vi "Read Hardware Interface State.vi"(8 "error in (no error)":errorcluster, 10 "hardware interface index":u16, 11 "PLBB in":refnum<class "PL BlackBox Modbus Client.lvclass">) -> (0 "error out":errorcluster, 2 "hardware interface state":T1, 3 "PLBB out":refnum<class "PL BlackBox Modbus Client.lvclass">)   [LabVIEW 2015, in "PL BlackBox Modbus Client.lvclass"]
doc: "Reads the hardware interface state."
uses:
  PL BlackBox Modbus Client.lvclass
  <vilib>/plasmapper/PL Modbus Client/PL Modbus Client.lvclass
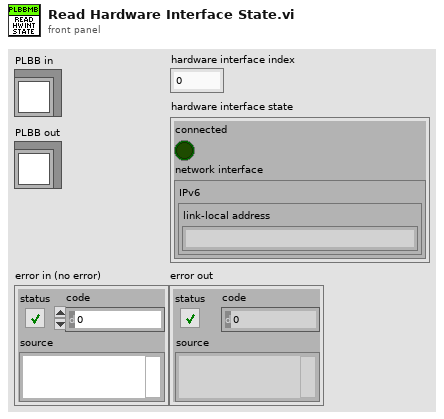
[diagram p1: front panel]
types:
  T1 = cluster{"connected":bool, "network interface":cluster{"IPv6":cluster{"link-local address":string}}}
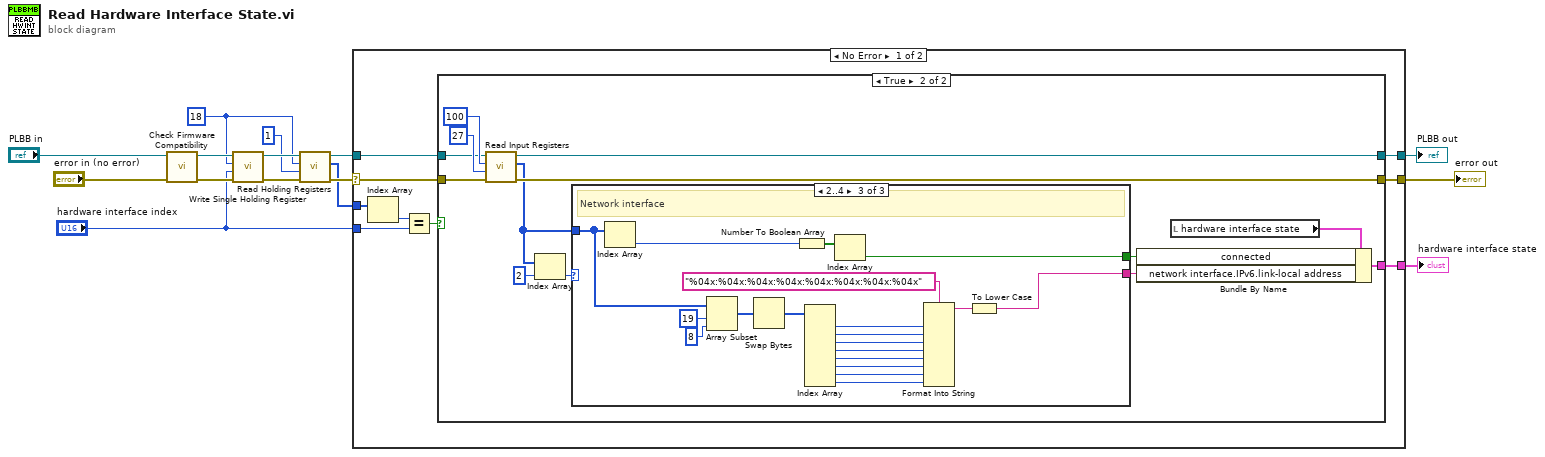
[diagram p0: block diagram]
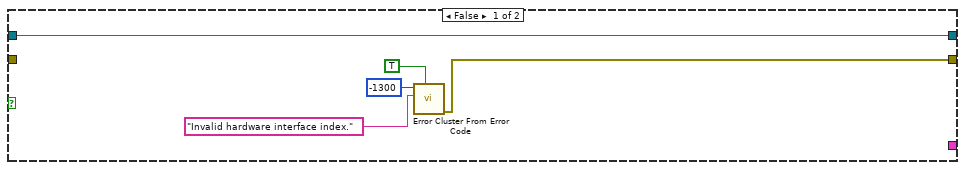
[diagram p2: hidden frame]
diagram:
  w7 = u16 18 ("address")
  n1 = call-dynamic "Check Firmware Compatibility.vi"("error in (no error)"="error in (no error)", "PLBB in"="PLBB in") -> ("error out"=w10:errorcluster, "PLBB out"=w11:refnum<class "PL BlackBox Modbus Client.lvclass">)  [unwired: 8 in]
  n2 = call <vilib>:"Write Single Holding Register.vi"("error in (no error)"=w10, "value"="hardware interface index", "address"=w7, "MODBUS in"=w11) -> ("error out"=w6:errorcluster, "MODBUS out"=w9:refnum<class "PL BlackBox Modbus Client.lvclass">)  [unwired: 6 in]
  n3 = call <vilib>:"Read Holding Registers.vi"("error in (no error)"=w6, "number of holding registers"=u16 1 ("address"), "address"=w7, "MODBUS in"=w9) -> ("error out"=w5:errorcluster, "values"=w3:u16[], "MODBUS out"=w4:refnum<class "PL BlackBox Modbus Client.lvclass">)  [unwired: 5 in]
  n4 = case shown="No Error" w5 {
    selector: w5 -> [w17 w62]
    tunnel: [w24 w62] -> w15
    tunnel: [w23 w63] -> w14
    tunnel: w4 -> [w18 w63]
    tunnel: w3 -> [w22 _]
    tunnel: "hardware interface index" -> [w20 _]
    tunnel: [w16 _] -> w1
    frame No Error {
      n5 = Index Array(array=w22) -> (element=w21:u16)  [unwired: 1 in]
      n6 = Equal?(x=w21, y=w20) -> (x = y?=w19:bool)
      n7 = case shown="True" w19 {
        tunnel: [w25 w32] -> w24
        tunnel: [w29 w33] -> w23
        tunnel: w18 -> [w29 w37]
        tunnel: w17 -> [_ w36]
        tunnel: [_ w41] -> w16
        frame False {
          n8 = call <vilib>:"Error Cluster From Error Code.vi"("show call chain? (False)"=TRUE, "error message (\"\")"="Invalid hardware interface index." ("error message (\"\")"), "error code (0)"=-1300) -> ("error out"=w25:errorcluster)  [unwired: 6 in]
        }
        frame True {
          n9 = call <vilib>:"Read Input Registers.vi"("error in (no error)"=w36, "number of input registers"=u16 27 ("address"), "address"=u16 100, "MODBUS in"=w37) -> ("error out"=w32:errorcluster, "values"=w30:u16[], "MODBUS out"=w33:refnum<class "PL BlackBox Modbus Client.lvclass">)  [unwired: 5 in]
          n10 = Index Array(array=w30, index=2) -> (element=w35:u16)
          n11 = case shown="2..4" w35 {
            tunnel: [_ _ w60] -> w40
            tunnel: w30 -> [_ _ w44]
            tunnel: [_ _ w53] -> w34
            frame 0, Default {
            }
            frame 1 {
              # "UART"
            }
            frame 2..4 {
              # "Network interface"
              n12 = Index Array(array=w44) -> (element=w59:u16)  [unwired: 1 in]
              n13 = Array Subset(array=w44, index=19, length=8) -> (w56:u16[])
              n14 = Swap Bytes(anything=w56) -> (byte swapped=w43:u16[])
              n15 = Number To Boolean Array(number=w59) -> (Boolean array=w61:bool[])
              n16 = Index Array(array=w43) -> (element #1=w52:u16, element #2=w51:u16, element #3=w50:u16, element #4=w49:u16, element #5=w48:u16, element #6=w47:u16, element #7=w46:u16, element #8=w45:u16)  [unwired: 8 in]
              n17 = Index Array(array=w61) -> (element=w60:bool)  [unwired: 1 in]
              n18 = Format Into String(format string="%04x:%04x:%04x:%04x:%04x:%04x:%04x:%04x", w52, w51, w50, w49, w48, w47, w46, w45) -> (resulting string=w54:string)  [unwired: 2 in, 1 out]
              n19 = To Lower Case(string=w54) -> (all lower case string=w53:string)
            }
          }
          n20 = local read "hardware interface state"() -> (w42:T1)
          n21 = Bundle By Name(cluster=w42, "connected"=w40, "network interface.IPv6.link-local address"=w34) -> (w41:T1)
        }
      }
    }
    frame Error {
    }
  }
  "error out" <- w15
  "PLBB out" <- w14
  "hardware interface state" <- w1
